vi "please_deer_god_3.vi"(0 "VISA resource name out":refnum<visa-resource-name>, 3 "error out 2":errorcluster) -> (6 "VISA resource name out 2":refnum<visa-resource-name>, 9 "error out":errorcluster)   [LabVIEW 2021]
panel:
  out "SCPI parameter input":string[](array[string])
  in  "secondary parameter":string(combo)="FUNCtion:impa D\n"
  in  "equivalent mode":string(combo)="FUNCtion:EQUivalent Pal\n"
  in  "voltage":string(combo)="VOLTage 0.6\n"
  in  "primary parameter":string(combo)="FUNCtion:impa C\n"
  in  "frequency":string(combo)="FREQuency\\s1000\\n"
  out "Parameters read for device":string[](array[string])
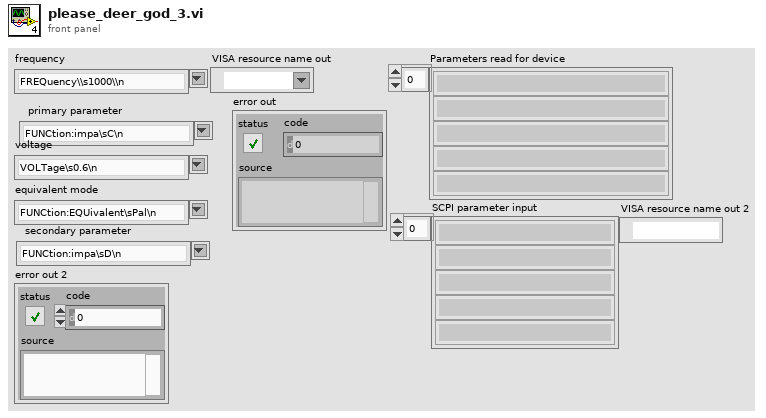
[diagram p1: front panel]
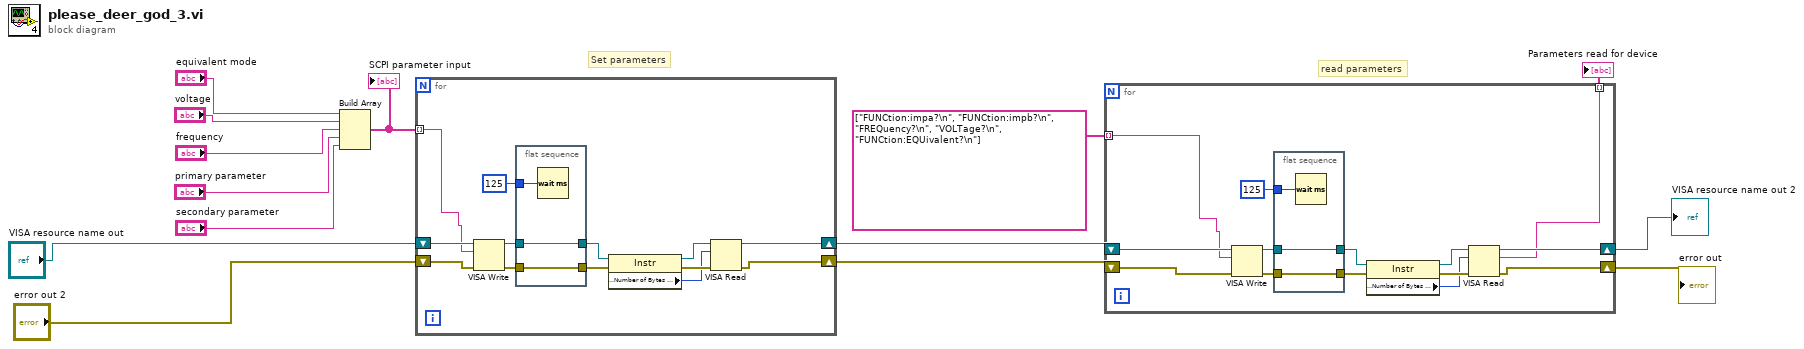
[diagram p0: block diagram]
diagram:
  # "read parameters"
  # "Set parameters"
  n1 = Build Array("equivalent mode", "voltage", "frequency", "primary parameter", "secondary parameter") -> (w10:string[])
  "SCPI parameter input" <- w10
  n2 = for {
    shift-right: [w19] -> w12
    shift-left: "VISA resource name out" -> [w20]
    shift-right: [w18] -> w11
    shift-left: "error out 2" -> [w15]
    tunnel: w10 -> [w16] mode=indexing
    n3 = VISA Write(VISA resource name=w20, write buffer=w16, error in (no error)=w15) -> (VISA resource name out=w25:refnum<visa-resource-name>, error out=w27:errorcluster)  [unwired: 1 out]
    n4 = flat-sequence {
      tunnel: w27 -> [w29]
      tunnel: [w29] -> w26
      tunnel: w25 -> [w28]
      tunnel: [w28] -> w24
      tunnel: u32 125 ("delay before read (ms)") -> [w30]
      frame #0 {
        n5 = Wait (ms)(milliseconds to wait=w30) -> ()  [unwired: 1 out]
      }
    }
    n6 = property class="Instr"(reference=w24, error in=w26) -> (reference out=w23:refnum<visa-resource-name>, error out=w22:errorcluster, "Serial Settings:Number of Bytes at Serial Port"=w21:u32)
    n7 = VISA Read(VISA resource name=w23, byte count=w21, error in (no error)=w22) -> (VISA resource name out=w19:refnum<visa-resource-name>, error out=w18:errorcluster)  [unwired: 2 out]
  }
  n8 = for {
    shift-right: [w35] -> w4
    shift-left: w12 -> [w37]
    shift-right: [w34] -> w3
    shift-left: w11 -> [w36]
    tunnel: string[] ["FUNCtion:impa?\n", "FUNCtion:impb?\n", "FREQuency?\n", "VOLTage?\n", "FUNCtion:EQUivalent?\n"] -> [w32] mode=indexing
    tunnel: [w31] -> w13 mode=indexing
    n9 = VISA Write(VISA resource name=w37, write buffer=w32, error in (no error)=w36) -> (VISA resource name out=w42:refnum<visa-resource-name>, error out=w44:errorcluster)  [unwired: 1 out]
    n10 = flat-sequence {
      tunnel: w44 -> [w46]
      tunnel: [w46] -> w43
      tunnel: w42 -> [w45]
      tunnel: [w45] -> w41
      tunnel: u32 125 ("delay before read (ms)") -> [w47]
      frame #0 {
        n11 = Wait (ms)(milliseconds to wait=w47) -> ()  [unwired: 1 out]
      }
    }
    n12 = property class="Instr"(reference=w41, error in=w43) -> (reference out=w40:refnum<visa-resource-name>, error out=w39:errorcluster, "Serial Settings:Number of Bytes at Serial Port"=w38:u32)
    n13 = VISA Read(VISA resource name=w40, byte count=w38, error in (no error)=w39) -> (VISA resource name out=w35:refnum<visa-resource-name>, read buffer=w31:string, error out=w34:errorcluster)  [unwired: 1 out]
  }
  "Parameters read for device" <- w13
  "VISA resource name out 2" <- w4
  "error out" <- w3
